vi "Stream Four Probe Asynchronous.vi"(10 "Error Stream gRPCid":T1, 11 "gRPCid":T1) -> ()   [LabVIEW 2019]
uses:
  VIs/MeasurementServer_gRPCid.ctl
  Global Operations.ctl
  VIs/labview-grpc-measurement-server.lvlib
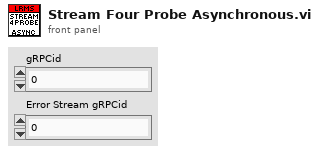
[diagram p1: front panel]
types:
  T1 = typedef "labview-grpc-measurement-server.lvlib/MeasurementServer_gRPCid.ctl" = u64
  T2 = typedef "Global Operations.ctl" = enum16{"Get", "Set"}
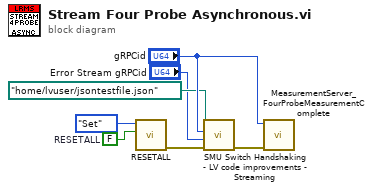
[diagram p0: block diagram]
diagram:
  w4 = FALSE  # RESETALL
  n1 = call "RESETALL.vi"("RESETALL"=w4, "Operation"=Global_Operations."Set") -> ("error out"=w2:errorcluster)  [unwired: 8 in, 1 out]
  n2 = call "SMU Switch Handshaking - LV code improvements - Streaming.vi"("error in"=w2, "Error Stream gRPCid"="Error Stream gRPCid", "gRPCid"="gRPCid", "file path (use dialog)"=path "/home/lvuser/jsontestfile.json") -> ("error out"=w5:errorcluster)  [unwired: 6 in, 1 out]
  n3 = call "MeasurementServer_FourProbeMeasurementComplete.vi"("gRPCid"="gRPCid", "error in (no error)"=w5) -> ()  [unwired: 8 in, 1 out]
